vi "ClosePopUpWindow.vi"() -> ()   [LabVIEW 2022 SP3]
panel:
  out "error out":errorcluster
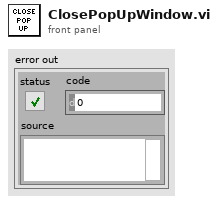
[diagram p1: front panel]
types:
  T1 = enum32{"Invalid", "Standard", "Closed", "Hidden", "Minimized", "Maximized"}
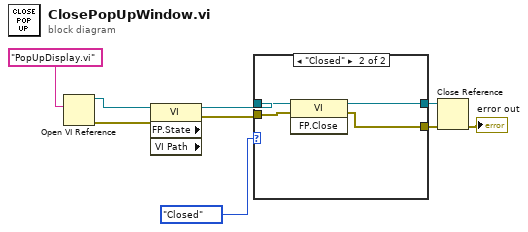
[diagram p0: block diagram]
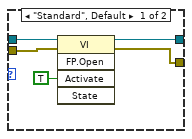
[diagram p2: hidden frame]
diagram:
  n1 = Open VI Reference(vi path="PopUpDisplay.vi" ("VI Name")) -> (vi reference=w3:refnum<vi>, error out=w2:errorcluster)  [unwired: 5 in]
  n2 = property class="VI" props=["FP.State", "VI Path"](reference=w3, error in=w2) -> (reference out=w8:refnum<vi>, error out=w7:errorcluster)  [unwired: 2 out]
  n3 = case shown="\"Closed\"" T1."Closed" ("Front Panel Window:State") {
    tunnel: [w11 w18] -> w9
    tunnel: w8 -> [w14 w17]
    tunnel: w7 -> [w12 w16]
    tunnel: [w13 w15] -> w6
    frame "Standard", Default {
      n4 = invoke class="VI" method="FP.Open"(reference=w14, error in=w12, "Activate"=TRUE ("Activate?")) -> (reference out=w13:refnum<vi>, error out=w11:errorcluster)  [unwired: 2 in, 3 out]
    }
    frame "Closed" {
      n5 = invoke class="VI" method="FP.Close"(reference=w17, error in=w16) -> (reference out=w15:refnum<vi>, error out=w18:errorcluster)  [unwired: 1 in, 1 out]
    }
  }
  n6 = Close Reference(reference=w6, error in (no error)=w9) -> (error out=→"error out":errorcluster)
